vi "refresh stuff.vi"(8 "error in (no error)":errorcluster, 11 "Waveform in":refnum<class "Waveform.lvclass">) -> (0 "error out":errorcluster, 3 "Waveform out":refnum<class "Waveform.lvclass">)   [LabVIEW 2012, in "Waveform.lvclass"]
uses:
  Waveform.lvclass
  Waveform.lvclass/Waveform.ctl
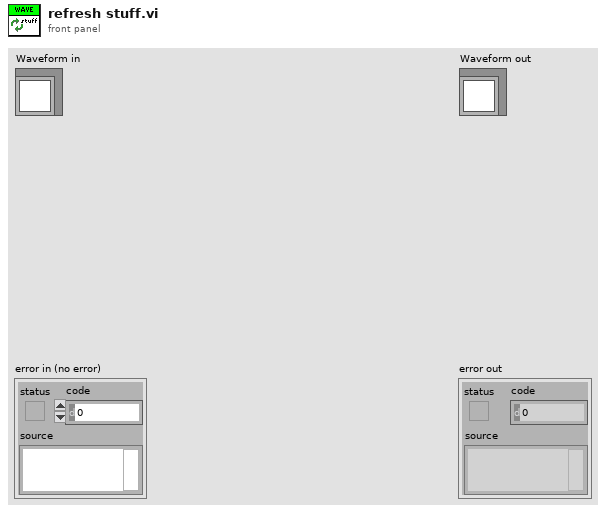
[diagram p1: front panel]
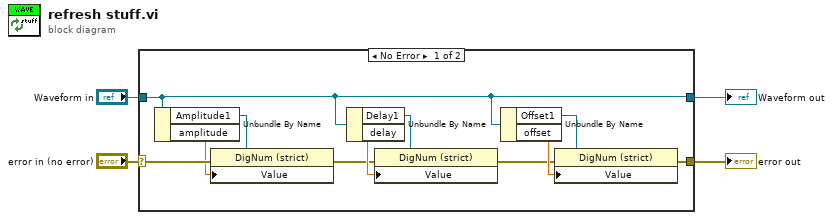
[diagram p0: block diagram]
diagram:
  n1 = case shown="No Error" "error in (no error)" {
    selector: "error in (no error)" -> [w15 w17]
    tunnel: [w5 w17] -> w3
    tunnel: [w8 w16] -> w1
    tunnel: "Waveform in" -> [w8 w16]
    frame No Error {
      n2 = Unbundle By Name(w8) -> ("Amplitude1"=w14:refnum<vi>, "amplitude"=w13:dbl[unit])
      n3 = property class="DigNum (strict)"(reference=w14, error in=w15, "Value"=w13) -> (error out=w7:errorcluster)  [unwired: 1 out]
      n4 = Unbundle By Name(w8) -> ("Delay1"=w11:refnum<vi>, "delay"=w12:dbl[unit])
      n5 = property class="DigNum (strict)"(reference=w11, error in=w7, "Value"=w12) -> (error out=w6:errorcluster)  [unwired: 1 out]
      n6 = Unbundle By Name(w8) -> ("Offset1"=w10:refnum<vi>, "offset"=w9:dbl[unit])
      n7 = property class="DigNum (strict)"(reference=w10, error in=w6, "Value"=w9) -> (error out=w5:errorcluster)  [unwired: 1 out]
    }
    frame Error {
    }
  }
  "error out" <- w3
  "Waveform out" <- w1
